vi "TREE_get tree-axis rev 1-0.vi"(8 "error in (no error)":errorcluster, 9 "allowed tree.axis IN":i32, 10 "Point IN":T1, 11 "tree.refNum IN":refnum<vi>) -> (0 "error out":errorcluster, 1 "current.axis OUT":i32, 2 "same tree.axis (T)":bool, 3 "tree.refNum OUT":refnum<vi>)   [LabVIEW 2014]
uses:
  <vilib>/Utility/miscctls.llb/LVPositionTypeDef.ctl
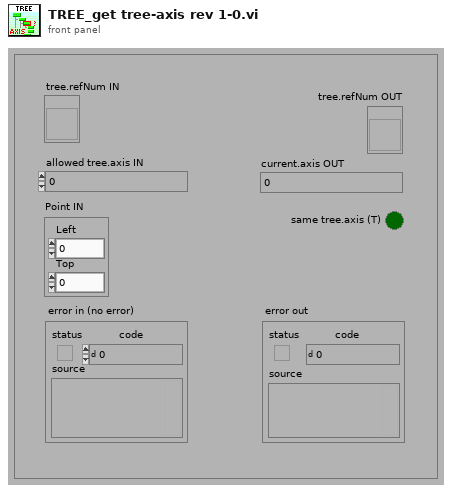
[diagram p1: front panel]
types:
  T1 = typedef "LVPositionTypeDef.ctl" = cluster{"Left":i32, "Top":i32}
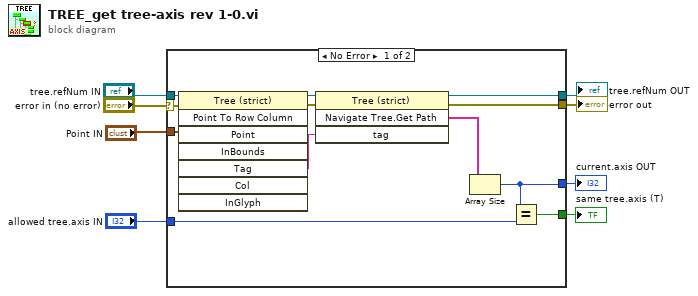
[diagram p0: block diagram]
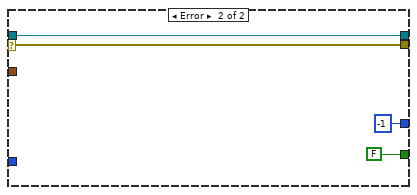
[diagram p2: hidden frame]
diagram:
  n1 = case shown="No Error" "error in (no error)" {
    selector: "error in (no error)" -> [w15 w23]
    tunnel: [w16 w23] -> w8
    tunnel: [w14 -1] -> w6
    tunnel: "tree.refNum IN" -> [w13 w22]
    tunnel: [w12 w22] -> w4
    tunnel: "allowed tree.axis IN" -> [w11 _]
    tunnel: [w10 FALSE] -> w2
    tunnel: "Point IN" -> [w9 _]
    frame No Error {
      n2 = invoke class="Tree (strict)" method="Point To Row Column"(reference=w13, error in=w15, "Point"=w9) -> (reference out=w20:refnum<vi>, error out=w19:errorcluster, "Tag"=w18:string)  [unwired: 5 in, 5 out]
      n3 = invoke class="Tree (strict)" method="Navigate Tree.Get Path"(reference=w20, error in=w19, "tag"=w18) -> (reference out=w12:refnum<vi>, error out=w16:errorcluster, "Navigate Tree:Get Path"=w17:string[])  [unwired: 1 in, 1 out]
      n4 = Array Size(array=w17) -> (size(s)=w14:i32)
      n5 = Equal?(x=w14, y=w11) -> (x = y?=w10:bool)
    }
    frame Error {
    }
  }
  "error out" <- w8
  "current.axis OUT" <- w6
  "tree.refNum OUT" <- w4
  "same tree.axis (T)" <- w2
